vi "FCT Request.vi"(8 "error in (no error)":errorcluster, 10 "Reqest":T1 {"Request" items=["Null Request"=0, "Request Parameter"=6, "Change Parameter"=8, "Request Lower Limit"=13, "Request Upper Limit"=14]}, 11 "FHPP in":refnum<class "FHPP.lvclass">) -> (0 "error out":errorcluster, 1 "Data":u32, 2 "Error Code":u32, 3 "FHPP Out":refnum<class "FHPP.lvclass">)   [LabVIEW 2022 SP3, in "FHPP.lvclass"]
doc: "Sends a FCT <b>Request</b> to the device. Waits for an answer. If transfer okay then <b>Data</b> is populated else <b>Error Code</b> gives the error code number of the error answer."
uses:
  FHPP.lvclass
  TypeDefs/FCT Request.ctl
  TypeDefs/ReqID.ctl
  TypeDefs/ResID.ctl
  FHPP.lvclass/FHPP.ctl
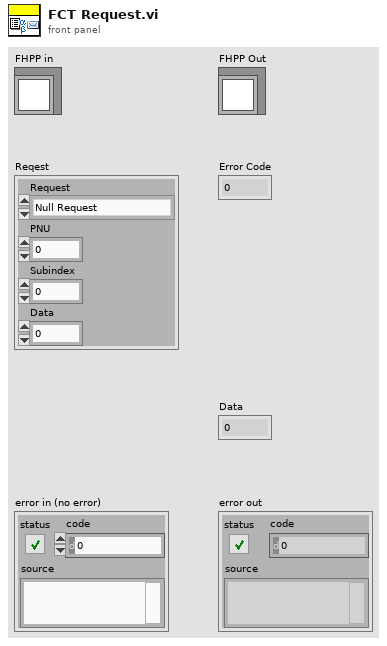
[diagram p1: front panel]
types:
  T1 = typedef "FHPP.lvclass/FCT Request.ctl" = cluster{"Request":T2, "PNU":u16, "Subindex":u16, "Data":u32}
  T2 = typedef "FHPP.lvclass/ReqID.ctl" = u8
  T3 = typedef "FHPP.lvclass/ResID.ctl" = u8
  T4 = typedef "FHPP.lvclass/FCT Response.ctl" = cluster{"ResID":T3, "PNU":u16, "Subindex":u16, "Data":u32}
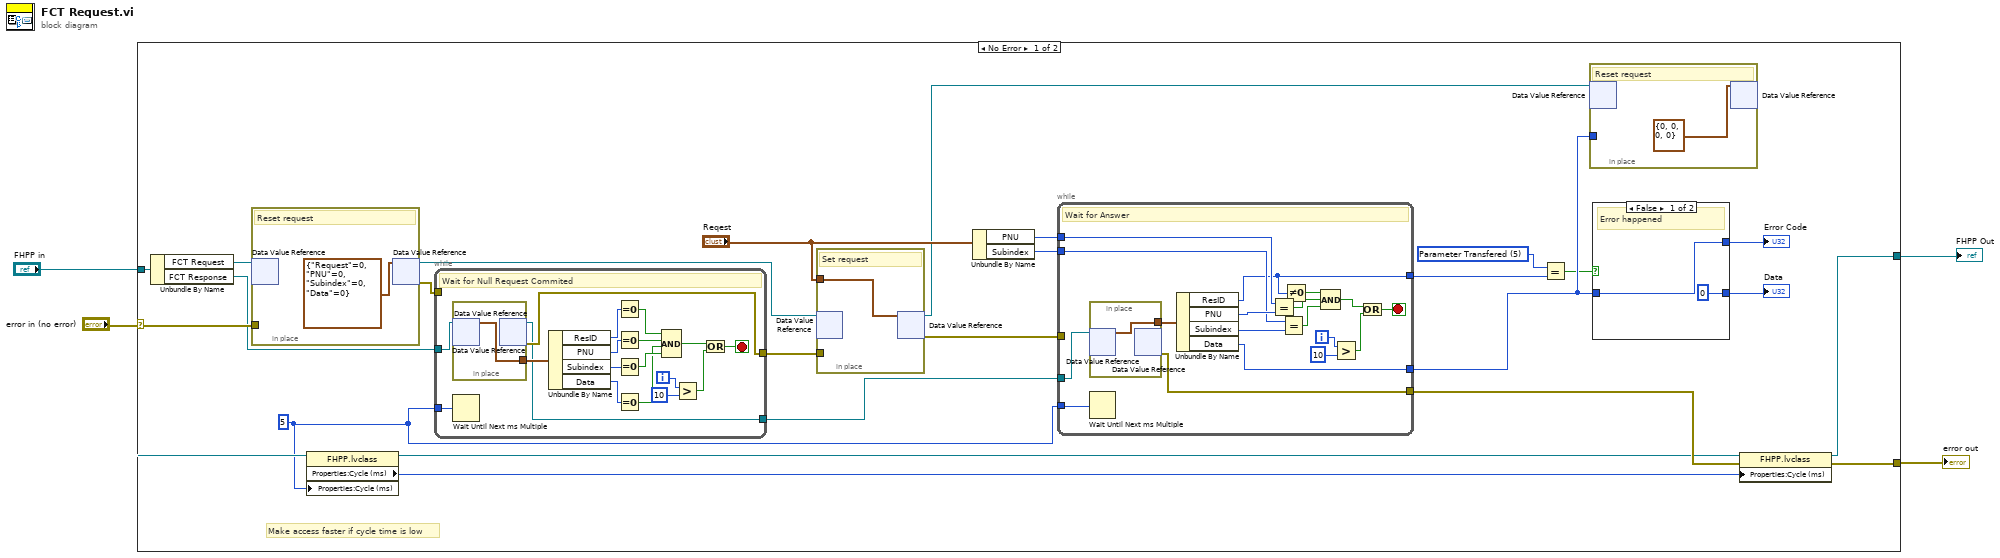
[diagram p0: block diagram]
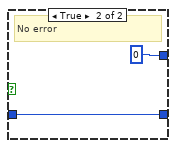
[diagram p2: hidden frame]
diagram:
  n1 = case shown="No Error" "error in (no error)" {
    selector: "error in (no error)" -> [w28 w76]
    tunnel: "FHPP in" -> [w10 w75]
    tunnel: [w6 w76] -> w2
    tunnel: [w5 w75] -> w1
    frame No Error {
      w9 = 5 ("Cycle (ms)")
      w23 = T3 5 items=["No Answer"=0, "Parameter Transfered"=5, "Error"=7] ("x")
      # "Make access faster if cycle time is low"
      n2 = Unbundle By Name(w10) -> ("FCT Request"=w12:refnum<data-value>, "FCT Response"=w13:refnum<data-value>)
      n3 = in-place {
        in-place-border: w28 -> [_]
        # "Reset request"
        n4 = in-place-dvr #1(w12) -> ()  [unwired: 2 out]
        n5 = in-place-dvr #1(T1 {"Request"=0, "PNU"=0, "Subindex"=0, "Data"=0} ("data value")) -> (w16:refnum<data-value>, w14:errorcluster)
      }
      n6 = property class="FHPP.lvclass"(reference=w10, "Properties:Cycle (ms)"=w9) -> (reference out=w7:refnum<class "FHPP.lvclass">, "Properties:Cycle (ms)"=w8:i32)  [unwired: 1 in, 1 out]
      n7 = while {
        tunnel: w13 -> [w70]
        tunnel: w9 -> [w69]
        tunnel: w14 -> [_]
        tunnel: [w54] -> w17
        tunnel: [w71] -> w18
        i -> [w67]
        stop <- w55 stop-if-true
        # "Wait for Null Request Commited"
        n8 = in-place {
          in-place-border: [w72] -> w61
          n9 = in-place-dvr #2(w70) -> (w72:T4)  [unwired: 1 out]
          n10 = in-place-dvr #2() -> (w54:refnum<data-value>, w71:errorcluster)  [unwired: 1 in]
        }
        n11 = Wait Until Next ms Multiple(millisecond multiple=w69) -> ()  [unwired: 1 out]
        n12 = Unbundle By Name(w61) -> ("ResID"=w63:T3, "PNU"=w62:u16, "Subindex"=w64:u16, "Data"=w65:u32)
        n13 = Equal To 0?(x=w63) -> (x = 0?=w58:bool)
        n14 = Equal To 0?(x=w62) -> (x = 0?=w57:bool)
        n15 = Equal To 0?(x=w64) -> (x = 0?=w60:bool)
        n16 = Equal To 0?(x=w65) -> (x = 0?=w59:bool)
        n17 = Compound Arithmetic op=AND(w58, w57, w59, w60) -> (w56:bool)
        n18 = Greater?(x=w67, y=10) -> (0:w66:bool)
        n19 = Or(x=w56, y=w66) -> (x .or. y?=w55:bool)
      }
      n20 = in-place {
        in-place-border: w18 -> [_]
        in-place-border: "Reqest" -> [w53]
        # "Set request"
        n21 = in-place-dvr #3(w16) -> ()  [unwired: 2 out]
        n22 = in-place-dvr #3(w53) -> (w11:refnum<data-value>, w15:errorcluster)
      }
      n23 = Unbundle By Name("Reqest") -> ("PNU"=w20:u16, "Subindex"=w21:u16)
      n24 = while {
        tunnel: w17 -> [w51]
        tunnel: w9 -> [w50]
        tunnel: w15 -> [_]
        tunnel: w20 -> [w41]
        tunnel: w21 -> [w38]
        tunnel: [w35] -> w22
        tunnel: [w37] -> w27
        tunnel: [w34] -> w29
        i -> [w48]
        stop <- w44 stop-if-true
        # "Wait for Answer"
        n25 = in-place {
          in-place-border: [w52] -> w46
          n26 = in-place-dvr #4(w51) -> (w52:T4)  [unwired: 1 out]
          n27 = in-place-dvr #4() -> (w34:errorcluster)  [unwired: 1 in, 1 out]
        }
        n28 = Wait Until Next ms Multiple(millisecond multiple=w50) -> ()  [unwired: 1 out]
        n29 = Unbundle By Name(w46) -> ("ResID"=w35:T3, "PNU"=w43:u16, "Subindex"=w40:u16, "Data"=w37:u32)
        n30 = Equal?(x=w41, y=w43) -> (x = y?=w42:bool)
        n31 = Equal?(x=w38, y=w40) -> (x = y?=w39:bool)
        n32 = Not Equal To 0?(x=w35) -> (x != 0?=w36:bool)
        n33 = Compound Arithmetic op=AND(w36, w42, w39) -> (w45:bool)
        n34 = Greater?(x=w48, y=10) -> (0:w47:bool)
        n35 = Or(x=w45, y=w47) -> (x .or. y?=w44:bool)
      }
      n36 = Equal?(x=w23, y=w22) -> (x = y?=w24:bool)
      n37 = in-place {
        in-place-border: w27 -> [_]
        # "Reset request"
        n38 = in-place-dvr #5(w11) -> ()  [unwired: 2 out]
        n39 = in-place-dvr #5(T1 {"Request"=0, "PNU"=0, "Subindex"=0, "Data"=0} ("data value")) -> ()  [unwired: 2 out]
      }
      n40 = case shown="False" w24 {
        tunnel: w27 -> [w30 w33]
        tunnel: [u32 0 ("Data") w33] -> w25
        tunnel: [w30 u32 0 ("Data")] -> w26
        frame False {
          # "Error happened"
        }
        frame True {
          # "No error"
        }
      }
      "Error Code" <- w26
      "Data" <- w25
      n41 = property class="FHPP.lvclass"(reference=w7, error in=w29, "Properties:Cycle (ms)"=w8) -> (reference out=w5:refnum<class "FHPP.lvclass">, error out=w6:errorcluster)
    }
    frame Error {
    }
  }
  "error out" <- w2
  "FHPP Out" <- w1
